vi "SetJSON.vi"(6 "Ignore if Not Found?":bool, 8 "Error In":errorcluster, 9 "Controls?":bool=TRUE, 10 "JSON Input":string, 11 "VI Refnum In":refnum<vi>) -> (0 "Error Out":errorcluster, 3 "VI Refnum Out":refnum<vi>)   [LabVIEW 2019, in "LabJSON.lvlib"]
doc: "Set JSON to controls for a given VI."
uses:
  LabJSON.lvlib
  aa3fc0e6-e883-47c7-bda4-2d6daf452595.vi
  <vilib>/JDP Science/JSONtext/JSON text to Variant.vi
  <vilib>/JDP Science/JSONtext/LVClass Serializer/JSONtext LVClass Serializer.lvclass
  <vilib>/JDP Science/JSONtext/JSONtext.lvlib
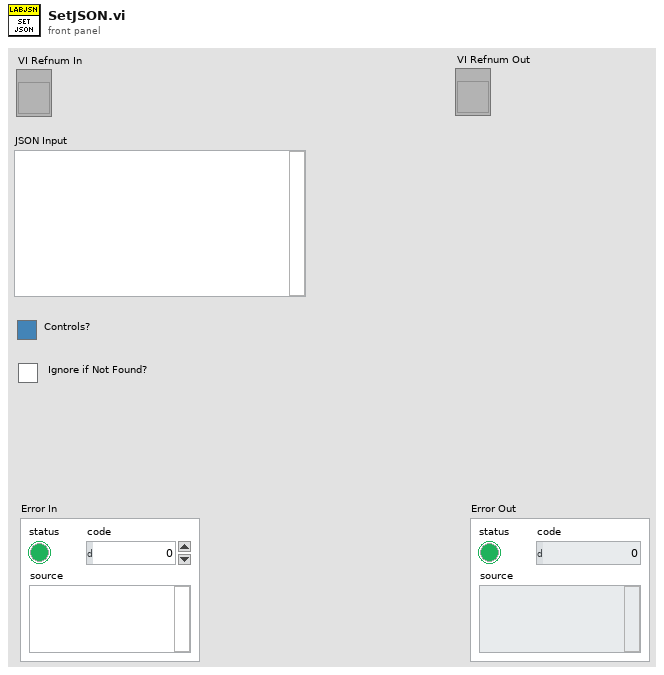
[diagram p1: front panel]
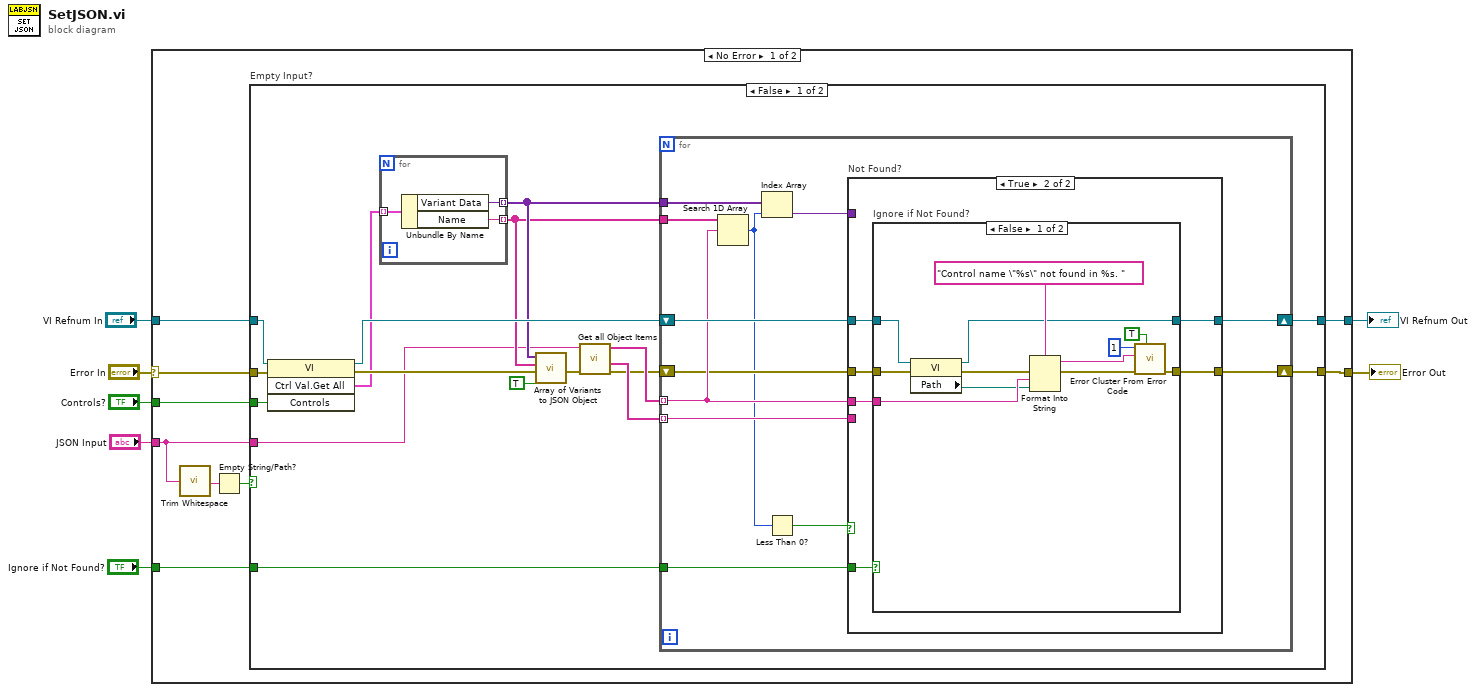
[diagram p0: block diagram]
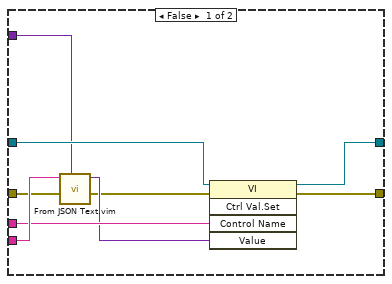
[diagram p2: hidden frame]
diagram:
  n1 = case shown="No Error" "Error In" {
    selector: "Error In" -> [w15 w81]
    tunnel: [w14 w81] -> w6
    tunnel: "JSON Input" -> [w11 _]
    tunnel: "VI Refnum In" -> [w16 w80]
    tunnel: [w13 w80] -> w3
    tunnel: "Controls?" -> [w12 _]
    tunnel: "Ignore if Not Found?" -> [w8 _]
    frame No Error {
      n2 = call <vilib>:"Trim Whitespace.vi"("string"=w11) -> ("trimmed string"=w9:string)  [unwired: 1 in]
      n3 = Empty String/Path?(string/path=w9) -> (empty?=w10:bool)
      n4 = case "Empty Input?" shown="False" w10 {
        tunnel: w16 -> [w23 w79]
        tunnel: w15 -> [w22 w78]
        tunnel: w11 -> [w21 _]
        tunnel: [w20 w78] -> w14
        tunnel: [w19 w79] -> w13
        tunnel: w12 -> [w18 _]
        tunnel: w8 -> [w17 _]
        frame False {
          n5 = invoke class="VI" method="Ctrl Val.Get All"(reference=w23, error in=w22, "Controls"=w18) -> (reference out=w33:refnum<vi>, error out=w32:errorcluster, "Get All Control Values Variant"=w25:cluster{"Name":string, "Variant Data":variant}[])  [unwired: 1 in, 1 out]
          n6 = for {
            tunnel: w25 -> [w36] mode=indexing
            tunnel: [w35] -> w27 mode=indexing
            tunnel: [w34] -> w26 mode=indexing
            n7 = Unbundle By Name(w36) -> ("Variant Data"=w35:variant, "Name"=w34:string)
          }
          n8 = call <vilib>:"Array of Variants to JSON Object.vi"("Pretty Print?"=TRUE, "error in (no error)"=w32, "Names"=w26, "Array"=w27) -> ("error out"=w28:errorcluster)  [unwired: 6 in, 1 out]
          n9 = call <vilib>:"Get all Object Items.vi"("error in (no error)"=w28, "JSON"=w21) -> ("error out"=w29:errorcluster, "<JSON>"=w30:string[], "Item Names"=w31:string[])  [unwired: 6 in, 1 out]
          n10 = for {
            shift-right: [w46] -> w19
            shift-left: w33 -> [w48]
            shift-right: [w47] -> w20
            shift-left: w29 -> [w40]
            tunnel: w31 -> [w41] mode=indexing
            tunnel: w30 -> [w42] mode=indexing
            tunnel: w26 -> [w45]
            tunnel: w27 -> [w44]
            tunnel: w17 -> [w37]
            n11 = Search 1D Array(1D array=w45, element=w41) -> (index of element=w39:i32)  [unwired: 1 in]
            n12 = Index Array(array=w44, index=w39) -> (element=w43:variant)
            n13 = Less Than 0?(x=w39) -> (x < 0?=w38:bool)
            n14 = case "Not Found?" shown="True" w38 {
              tunnel: w48 -> [w57 w59]
              tunnel: [w56 w62] -> w47
              tunnel: [w55 w58] -> w46
              tunnel: w43 -> [w54 _]
              tunnel: w42 -> [w53 _]
              tunnel: w41 -> [w52 w61]
              tunnel: w40 -> [w50 w63]
              tunnel: w37 -> [_ w60]
              frame False {
                n15 = call "From JSON Text.vim"("Data Type and Default Value"=w54, "error in (no error)"=w50, "JSON"=w53) -> ("error out"=w49:errorcluster, "Data out"=w51:variant)  [unwired: 7 in]
                n16 = invoke class="VI" method="Ctrl Val.Set"(reference=w57, error in=w49, "Control Name"=w52, "Value"=w51) -> (reference out=w55:refnum<vi>, error out=w56:errorcluster)  [unwired: 1 in, 3 out]
              }
              frame True {
                n17 = case "Ignore if Not Found?" shown="False" w60 {
                  tunnel: w63 -> [w68 w77]
                  tunnel: [w75 w77] -> w62
                  tunnel: w61 -> [w70 _]
                  tunnel: w59 -> [w67 w76]
                  tunnel: [w64 w76] -> w58
                  frame False {
                    n18 = property class="VI"(reference=w67, error in=w68) -> (reference out=w64:refnum<vi>, error out=w65:errorcluster, "Path"=w66:path)
                    n19 = Format Into String(format string="Control name \"%s\" not found in %s. ", error in=w65, w70, w66) -> (resulting string=w69:string, error out=w72:errorcluster)  [unwired: 1 in]
                    n20 = call <vilib>:"Error Cluster From Error Code.vi"("show call chain? (False)"=TRUE, "error in (no error)"=w72, "error message (\"\")"=w69, "error code (0)"=1) -> ("error out"=w75:errorcluster)  [unwired: 5 in]
                  }
                  frame True {
                    # "Ignore"
                  }
                }
              }
            }
          }
        }
        frame True {
          # "No Action Needed"
        }
      }
    }
    frame Error {
    }
  }
  "Error Out" <- w6
  "VI Refnum Out" <- w3
